vi "TRAJECTORY_EXECUTE_W_EST.vi"(6 "RamseteEnable":bool=TRUE, 8 "Init":bool, 9 "Input Sensors":T5, 10 "Max Speed\nFT/SEC":dbl, 11 "Wheel Base FT":dbl) -> (0 "AtReference":bool, 1 "Right Speed Target":dbl, 2 "Left Speed Target":dbl, 3 "outRAMSETE (SI)":T7={"B"=2.0, "Zeta"=0.7, "poseTolerance"={"TRANSLATION"={"X"=0.0, "Y"=0.0}, "ROTATION"={"VALUE"=0.0, "COS"=1.0, "SIN"=0.0}}, "poseError"={"TRANSLATION"={"X"=0.0, "Y"=0.0}, "ROTATION"={"VALUE"=0.0, "COS"=1.0, "SIN"=0.0}}, "Enabled"=TRUE} {"poseError"."ROTATION"."SIN" format="%13.4f"; "poseError"."ROTATION"."COS" format="%13.4f"; "poseError"."ROTATION"."VALUE" format="%13.4f"; "poseError"."TRANSLATION"."Y" format="%14.3f"; "poseError"."TRANSLATION"."X" format="%14.3f"; "poseTolerance"."ROTATION"."SIN" format="%13.4f"; "poseTolerance"."ROTATION"."COS" format="%13.4f"; "poseTolerance"."ROTATION"."VALUE" format="%13.4f"; "poseTolerance"."TRANSLATION"."Y" format="%14.3f"; "poseTolerance"."TRANSLATION"."X" format="%14.3f"; "Zeta" format="%12.3f"; "B" format="%12.3f"}, 4 "OutputTRAJ_STATE (SI)":T6={"TimeSeconds"=0.0, "Velocity"=0.0, "Acceleration"=0.0, "POSE"={"TRANSLATION"={"X"=0.0, "Y"=0.0}, "ROTATION"={"VALUE"=0.0, "COS"=1.0, "SIN"=0.0}}, "Curvature"=0.0} {"POSE"."ROTATION"."SIN" format="%13.4f"; "POSE"."ROTATION"."COS" format="%13.4f"; "POSE"."ROTATION"."VALUE" format="%13.4f"; "POSE"."TRANSLATION"."Y" format="%14.3f"; "POSE"."TRANSLATION"."X" format="%14.3f"}, 5 "Odom Pose Est Diff":T4={"TRANSLATION"={"X"=0.0, "Y"=0.0}, "ROTATION"={"VALUE"=0.0, "COS"=1.0, "SIN"=0.0}} {"ROTATION"."SIN" format="%13.4f"; "ROTATION"."COS" format="%13.4f"; "ROTATION"."VALUE" format="%13.4f"; "TRANSLATION"."Y" format="%14.3f"; "TRANSLATION"."X" format="%14.3f"}, 7 "Pose Est Info":cluster{"Estimated Pose":T1, "Error":bool} {"Estimated Pose"."ROTATION"."SIN" format="%13.4f"; "Estimated Pose"."ROTATION"."COS" format="%13.4f"; "Estimated Pose"."ROTATION"."VALUE" format="%13.4f"; "Estimated Pose"."TRANSLATION"."Y" format="%14.3f"; "Estimated Pose"."TRANSLATION"."X" format="%14.3f"})   [LabVIEW 2019]
uses:
  <vilib>/Rock Robotics/WPI/ThirdParty/JAS_Junk/TrajLib/RAMSETE.ctl
  <vilib>/Rock Robotics/WPI/ThirdParty/JAS_Junk/TrajLib/POSE2D.ctl
  <vilib>/Rock Robotics/WPI/ThirdParty/JAS_Junk/TrajLib/TRANSLATION2D.ctl
  <vilib>/Rock Robotics/WPI/ThirdParty/JAS_Junk/TrajLib/ROTATION2D.ctl
  <vilib>/Rock Robotics/WPI/ThirdParty/JAS_Junk/TrajLib/TRAJ_STATE.ctl
  TRAJ_EXEC_INPUT_SENSORS.ctl
  <vilib>/Rock Robotics/WPI/ThirdParty/JAS_Junk/TrajLib/TRANSFORM2D.ctl
  <vilib>/Rock Robotics/WPI/ThirdParty/JAS_Junk/TrajLib/Rotation_CreateAngle.vi
  <vilib>/Rock Robotics/WPI/ThirdParty/JAS_Junk/TrajLib/Translation_Create.vi
  <vilib>/Rock Robotics/WPI/ThirdParty/JAS_Junk/TrajLib/Pose_RelativeTo.vi
  <vilib>/Rock Robotics/WPI/ThirdParty/JAS_Junk/TrajLib/Transform_Create_TransRot.vi
  <vilib>/Rock Robotics/WPI/ThirdParty/JAS_Junk/TrajLib/Transform_Create_PosePose.vi
  <vilib>/Rock Robotics/WPI/ThirdParty/JAS_Junk/TrajLib/Pose_New_TRRO.vi
  <vilib>/Rock Robotics/WPI/ThirdParty/JAS_Junk/TrajLib/Rotation_UnaryMinus.vi
  <vilib>/Rock Robotics/WPI/ThirdParty/JAS_Junk/TrajLib/Translation_RotateBy.vi
  <vilib>/Rock Robotics/WPI/ThirdParty/JAS_Junk/TrajLib/Translation_Minus.vi
  <vilib>/Rock Robotics/WPI/ThirdParty/JAS_Junk/TrajLib/Rotation_Minus.vi
  <vilib>/Rock Robotics/WPI/ThirdParty/JAS_Junk/TrajLib/Rotation_RotateBy.vi
  <vilib>/Rock Robotics/WPI/ThirdParty/JAS_Junk/TrajLib/Rotation_CreateXY.vi
  <vilib>/Rock Robotics/WPI/ThirdParty/JAS_Junk/TrajLib/Util_CalcDist.vi
  <vilib>/Rock Robotics/WPI/ThirdParty/JAS_Junk/TrajLib/Trajectory_Library.lvlib
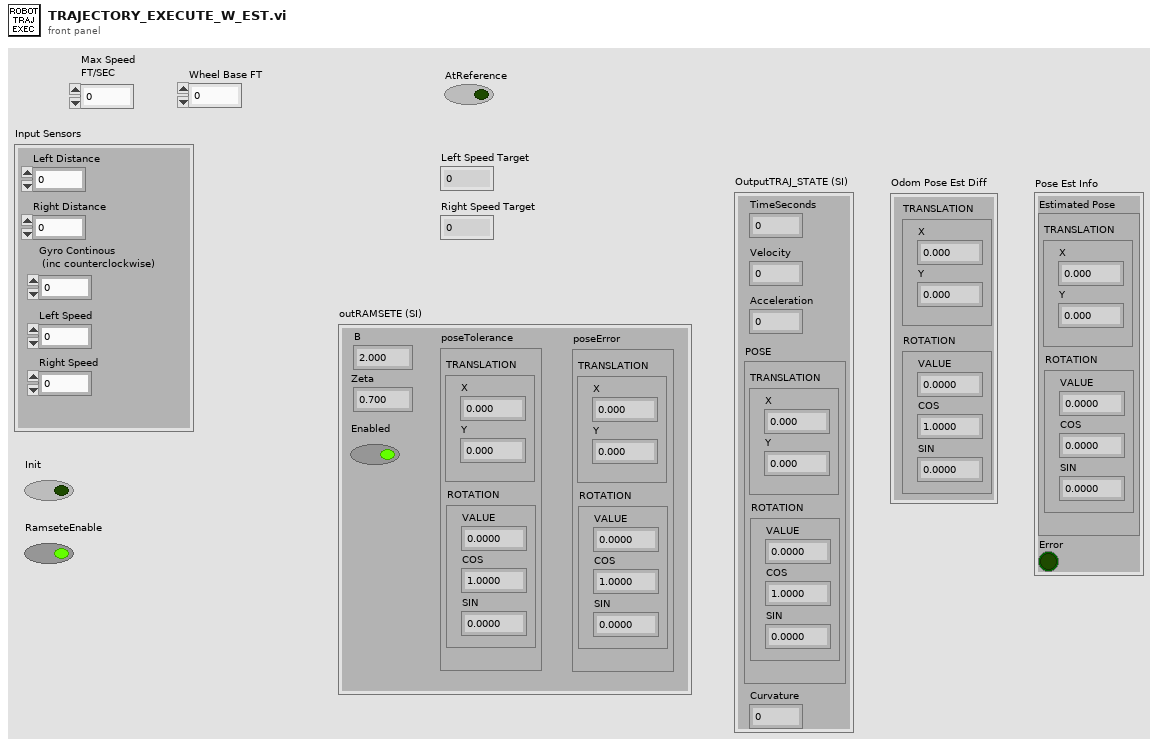
[diagram p1: front panel]
types:
  T1 = typedef "Trajectory_Library.lvlib/POSE2D.ctl" = cluster{"TRANSLATION":T2, "ROTATION":T3}
  T2 = typedef "Trajectory_Library.lvlib/TRANSLATION2D.ctl" = cluster{"X":dbl, "Y":dbl}
  T3 = typedef "Trajectory_Library.lvlib/ROTATION2D.ctl" = cluster{"VALUE":dbl, "COS":dbl, "SIN":dbl}
  T4 = typedef "Trajectory_Library.lvlib/TRANSFORM2D.ctl" = cluster{"TRANSLATION":T2, "ROTATION":T3}
  T5 = typedef "TRAJ_EXEC_INPUT_SENSORS.ctl" = cluster{"Left Distance":dbl, "Right Distance":dbl, "Gyro Continous\n (inc counterclockwise)":dbl, "Left Speed":dbl, "Right Speed":dbl}
  T6 = typedef "Trajectory_Library.lvlib/TRAJ_STATE.ctl" = cluster{"TimeSeconds":dbl, "Velocity":dbl, "Acceleration":dbl, "POSE":T1, "Curvature":dbl}
  T7 = typedef "Trajectory_Library.lvlib/RAMSETE.ctl" = cluster{"B":dbl, "Zeta":dbl, "poseTolerance":T1, "poseError":T1, "Enabled":bool}
  T8 = typedef "Trajectory_Library.lvlib/DIFF_DRIVE_POSE_EST.ctl" = cluster{"M_VisionDiscR":T9, "m_nominal_dT":dbl, "m_PrevTime_Sec":dbl, "m_GyroOffset":T3, "m_PrevAngle":T3, "StartLeftEnc_M":dbl, "StartRightEnc_M":dbl, "m_Observer":T10, "m_latencyCompensator":T13}
  T9 = typedef "NI_Matrix.lvlib/RealMatrix.ctl" = dbl[][]
  T10 = typedef "Trajectory_Library.lvlib/UNSCENTED_KALMAN_FILTER.ctl" = cluster{"m_P":T9, "m_xHat":T9, "States":i32, "Outputs":i32, "m_ContR":T9, "m_ContQ":T9, "m_SigmasF":T9, "m_dT_Sec":dbl, "MERWE_SCALED_SIGMA_PTS":T11, "meanFuncX":T12, "meanFuncY":T12, "residualFuncX":T12, "residualFuncY":T12, "addFuncX":T12, "addFuncXExtra":variant, "residualFuncYExtra":variant, "residualFuncXExtra":variant, "MeanFuncYExtra":variant, "MeanFuncXExtra":variant, "Inputs":i32}
  T11 = typedef "Trajectory_Library.lvlib/MERWE_SCALED_SIGMA_PTS.ctl" = cluster{"m_Wm":T9, "States":i32, "Alpha":dbl, "m_Wc":T9, "Kappa":i32}
  T12 = typedef "Trajectory_Library.lvlib/BiFun_Matrix_FUNC_TYPE.ctl" = refnum<vi>
  T13 = typedef "Trajectory_Library.lvlib/KALMAN_FILTER_LATENCY_COMP.ctl" = cluster{"m_pastObserverSnapshots ":T14[]}
  T14 = typedef "Trajectory_Library.lvlib/OBSERVER_SNAP_LIST_ITEM.ctl" = cluster{"TimeStamp":dbl, "OBSERVER_SNAPSHOT":T15}
  T15 = typedef "Trajectory_Library.lvlib/OBSERVER_SNAPSHOT.ctl" = cluster{"ErrorCoVariance":T9, "xHat":T9, "LocalMeasurements":T9, "Inputs":T9}
  T16 = typedef "Trajectory_Library.lvlib/TRAJECTORY.ctl" = cluster{"TotalTImeSecs":dbl, "States":T6[]}
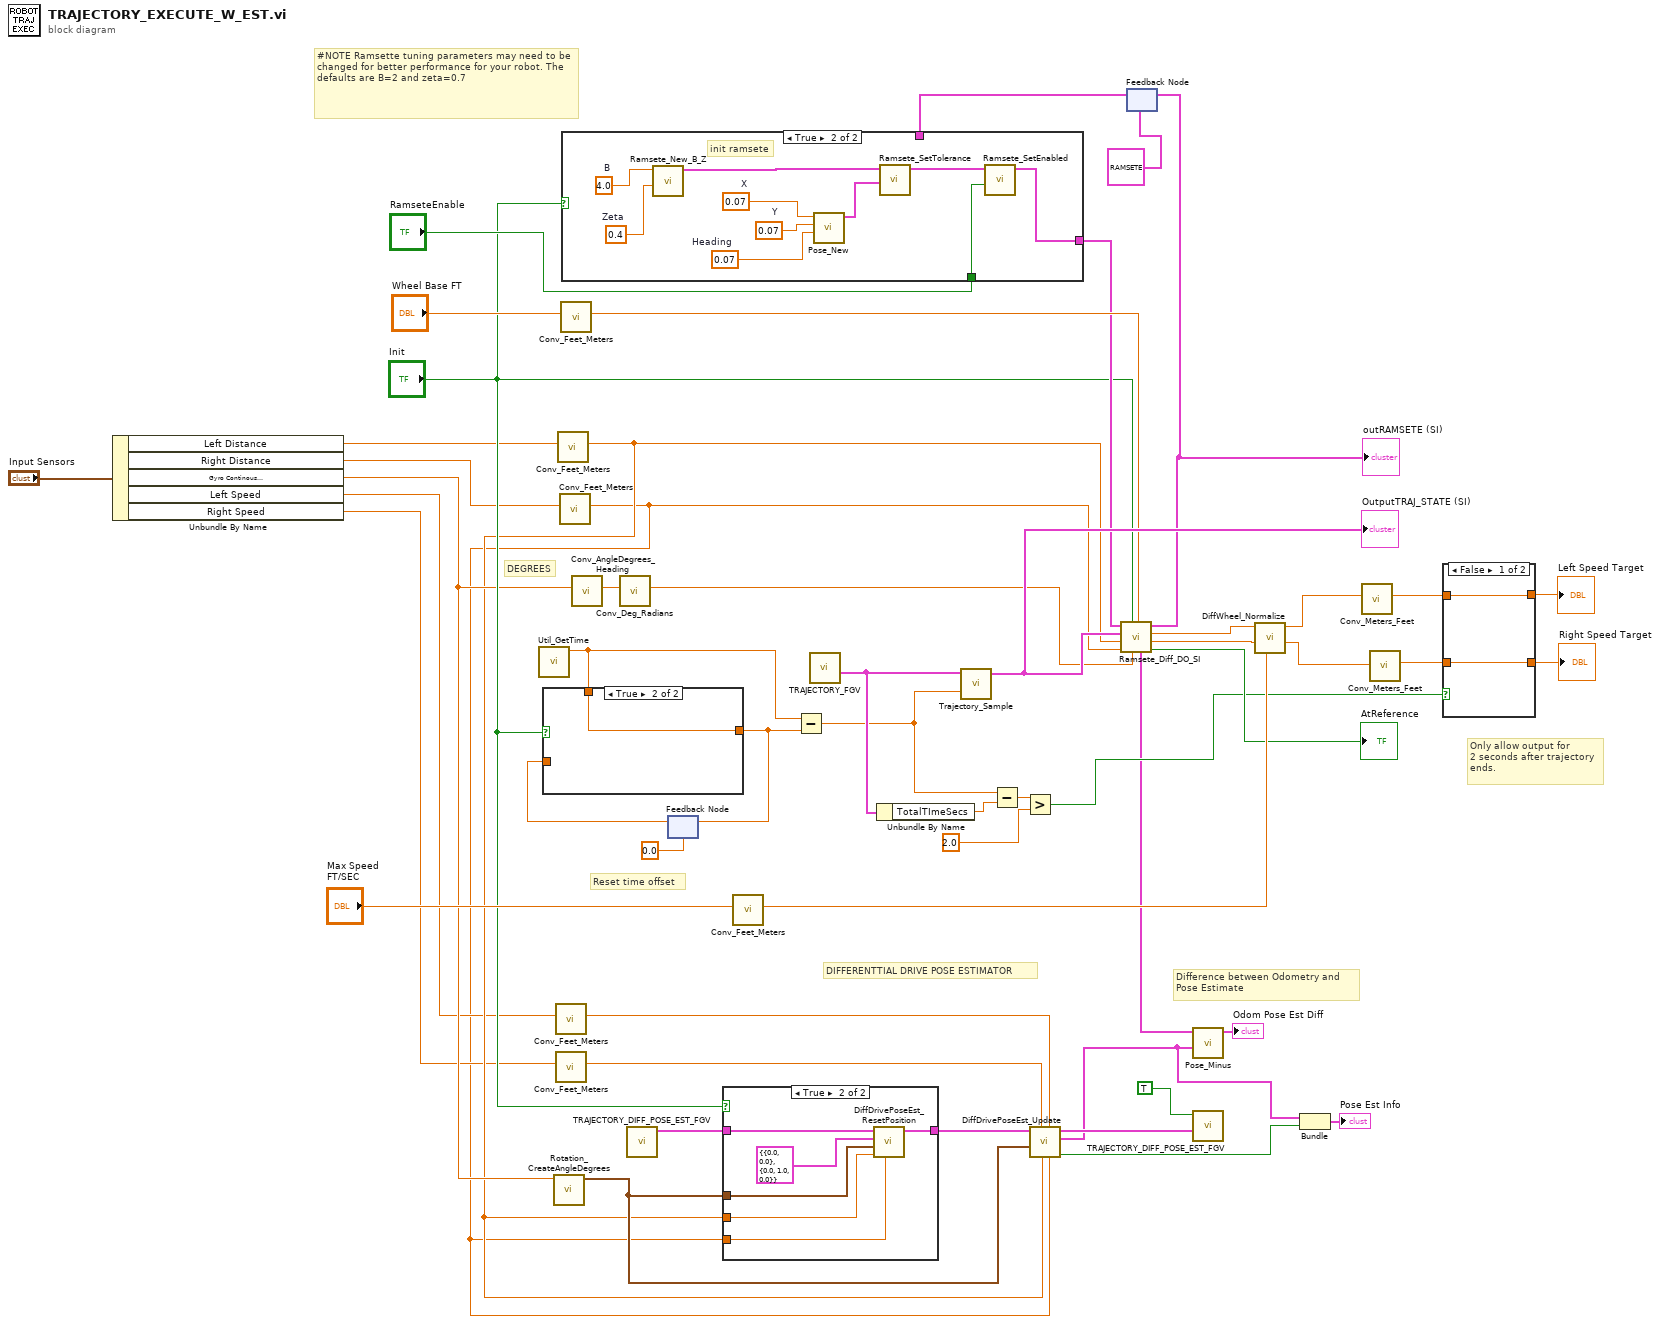
[diagram p0: block diagram]
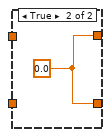
[diagram p4: hidden frame]
diagram:
  # "Difference between Odometry and\nPose Estimate"
  # "DIFFERENTTIAL DRIVE POSE ESTIMATOR"
  # "DEGREES"
  # "#NOTE Ramsette tuning parameters may need to be changed for better performance for your robot. The defaults are B=2 and zeta=0.7"
  # "Only allow output for\n2 seconds after trajectory\nends."
  # "Reset time offset"
  n1 = Unbundle By Name("Input Sensors") -> ("Left Distance"=w14:dbl, "Right Distance"=w13:dbl, "Gyro Continous\n (inc counterclockwise)"=w12:dbl, "Left Speed"=w10:dbl, "Right Speed"=w9:dbl)
  n2 = call <vilib>:"Util_GetTime.vi"() -> ("FPGA_Time_Seconds"=w23:dbl)  [unwired: 10 in, 1 out]
  n3 = call <vilib>:"Rotation_CreateAngleDegrees.vi"("Angle_Degrees"=w12) -> ("ROTATION"=w16:T3)  [unwired: 10 in]
  n4 = call <vilib>:"Conv_Feet_Meters.vi"("Feet"=w10) -> ("Meters"=w8:dbl)  [unwired: 10 in]
  n5 = call <vilib>:"Conv_Feet_Meters.vi"("Feet"=w9) -> ("Meters"=w7:dbl)  [unwired: 10 in]
  n6 = call <vilib>:"Conv_Feet_Meters.vi"("Feet"=w14) -> ("Meters"=w11:dbl)  [unwired: 10 in]
  n7 = call <vilib>:"Conv_Feet_Meters.vi"("Feet"=w13) -> ("Meters"=w4:dbl)  [unwired: 10 in]
  n8 = call <vilib>:"Conv_Feet_Meters.vi"("Feet"="Wheel Base FT") -> ("Meters"=w28:dbl)  [unwired: 10 in]
  n9 = call <vilib>:"Conv_AngleDegrees_Heading.vi"("Degrees"=w12) -> ("Heading Degrees"=w41:dbl)  [unwired: 10 in]
  n10 = call <vilib>:"Conv_Deg_Radians.vi"("Degress"=w41) -> ("Radians"=w29:dbl)  [unwired: 10 in]
  n11 = call "TRAJECTORY_DIFF_POSE_EST_FGV.vi"() -> ("out DIFF_DRIVE_POSE_EST 2"=w19:T8)  [unwired: 11 in]
  n12 = feedback #1(0.0 ("TIME")) -> (w51:dbl)
  n13 = case shown="True" "Init" {
    tunnel: [w53 w54] -> w50
    tunnel: w51 -> [w53 _]
    tunnel: w23 -> [_ w54]
    frame False {
    }
    frame True {
    }
  }
  n14 = feedback-in #1(w50) -> ()
  n15 = case shown="True" "Init" {
    tunnel: w19 -> [w55 w61]
    tunnel: [w55 w60] -> w18
    tunnel: w11 -> [_ w59]
    tunnel: w4 -> [_ w58]
    tunnel: w16 -> [_ w56]
    frame False {
    }
    frame True {
      n16 = call <vilib>:"DiffDrivePoseEst_ResetPosition.vi"("RightDistance_M"=w58, "LeftDistance_M"=w59, "Gyro"=w56, "Pose"=T1 {"TRANSLATION"={"X"=0.0, "Y"=0.0}, "ROTATION"={"VALUE"=0.0, "COS"=1.0, "SIN"=0.0}}, "in DiffDrivePoseEstimate"=w61) -> ("Out DiffDrivePoseEstimate"=w60:T8)  [unwired: 6 in]
    }
  }
  n17 = call <vilib>:"Conv_Feet_Meters.vi"("Feet"="Max Speed\nFT/SEC") -> ("Meters"=w45:dbl)  [unwired: 10 in]
  n18 = Subtract(x=w23, y=w50) -> (x-y=w38:dbl)
  n19 = call "TRAJECTORY_FGV.vi"() -> ("outTRAJECTORY"=w40:T16)  [unwired: 11 in]
  n20 = Unbundle By Name(w40) -> ("TotalTImeSecs"=w39:dbl)
  n21 = call <vilib>:"Trajectory_Sample.vi"("Time"=w38, "InputTRAJECTORY"=w40) -> ("OutputTRAJ_STATE"=w30:T6)  [unwired: 9 in]
  "OutputTRAJ_STATE (SI)" <- w30
  n22 = Subtract(x=w38, y=w39) -> (x-y=w37:dbl)
  n23 = Greater?(x=w37, y=2.0) -> (0:w35:bool)
  n24 = call <vilib>:"DiffDrivePoseEst_Update.vi"("RightDistance"=w4, "LeftSpeed"=w8, "LeftDistance"=w11, "RightSpeed"=w7, "GyroAngle"=w16, "in DiffDrivePoseEstimate"=w18) -> ("Error"=w2:bool, "Estimated Pose"=w3:T1, "Out DiffDrivePoseEstimate"=w17:T8)  [unwired: 3 in]
  n25 = feedback #2(T7 {"B"=2.0, "Zeta"=0.7, "poseTolerance"={"TRANSLATION"={"X"=0.0, "Y"=0.0}, "ROTATION"={"VALUE"=0.0, "COS"=1.0, "SIN"=0.0}}, "poseError"={"TRANSLATION"={"X"=0.0, "Y"=0.0}, "ROTATION"={"VALUE"=0.0, "COS"=1.0, "SIN"=0.0}}, "Enabled"=TRUE} ("RAMSETE")) -> (w26:T7)
  n26 = case shown="True" "Init" {
    tunnel: w26 -> [w62 _]
    tunnel: [w62 w70] -> w25
    tunnel: "RamseteEnable" -> [_ w63]
    frame False {
    }
    frame True {
      w64 = 0.4  # Zeta
      w65 = 4.0  # B
      w66 = 0.07  # Heading
      w67 = 0.07  # Y
      w68 = 0.07  # X
      # "init ramsete"
      n27 = call <vilib>:"Ramsete_New_B_Z.vi"("Zeta"=w64, "B"=w65) -> ("outRAMSETE"=w72:T7)  [unwired: 9 in]
      n28 = call <vilib>:"Pose_New.vi"("Heading"=w66, "Y"=w67, "X"=w68) -> ("out POSe"=w69:T1)  [unwired: 8 in]
      n29 = call <vilib>:"Ramsete_SetTolerance.vi"("tolerancePose"=w69, "inRAMSETE"=w72) -> ("outRAMSETE"=w71:T7)  [unwired: 9 in]
      n30 = call <vilib>:"Ramsete_SetEnabled.vi"("Enabled"=w63, "inRAMSETE"=w71) -> ("outRAMSETE"=w70:T7)  [unwired: 9 in]
    }
  }
  n31 = call <vilib>:"Ramsete_Diff_DO_SI.vi"("WheelBase-Meters"=w28, "Gyro-Radians"=w29, "Reset"="Init", "RightDist-Meters"=w4, "LeftDist-Meters"=w11, "TRAJ_STATE"=w30, "inRAMSETE"=w25) -> ("AtReference"=→"AtReference":bool, "RightVelDmd"=w46:dbl, "LeftVelDmd"=w47:dbl, "outRAMSETE"=w27:T7, "CurrentRelativePose"=w6:T1)
  "outRAMSETE (SI)" <- w27
  n32 = feedback-in #2(w27) -> ()
  n33 = call <vilib>:"Pose_Minus.vi"("other TRANSFORM"=w3, "in POSE"=w6) -> ("outTRANSFORM"=→"Odom Pose Est Diff":T4)  [unwired: 9 in]
  n34 = call "TRAJECTORY_DIFF_POSE_EST_FGV.vi"("IN DIFF_DRIVE_POSE_EST"=w17, "WRITE"=TRUE) -> ()  [unwired: 9 in, 1 out]
  n35 = call <vilib>:"DiffWheel_Normalize.vi"("Max Speed"=w45, "Right Wheel Demand"=w46, "Left Wheel Demand"=w47) -> ("Normalized Right Wheel Demand"=w42:dbl, "Normalized Left Wheel Demand"=w43:dbl)  [unwired: 7 in]
  n36 = Bundle("Estimated Pose"=w3, "Error"=w2) -> (→"Pose Est Info":cluster{"Estimated Pose":T1, "Error":bool})  [unwired: 1 in]
  n37 = call <vilib>:"Conv_Meters_Feet.vi"("Meters"=w43) -> ("Feet"=w32:dbl)  [unwired: 10 in]
  n38 = call <vilib>:"Conv_Meters_Feet.vi"("Meters"=w42) -> ("Feet"=w31:dbl)  [unwired: 10 in]
  n39 = case shown="False" w35 {
    tunnel: [w74 w75] -> w34
    tunnel: [w73 w75] -> w33
    tunnel: w32 -> [w74 _]
    tunnel: w31 -> [w73 _]
    frame False {
    }
    frame True {
      w75 = 0.0
    }
  }
  "Left Speed Target" <- w34
  "Right Speed Target" <- w33
